vi "GUI Monitoring Graph Selection Window.vi"(14 "OK Button":bool) -> (4 "Graph Selector Out":T1[](array[typedef])=[{"Name"="BPMs Horizontais", "Active"=TRUE}, {"Name"="BPMs Verticais", "Active"=TRUE}, {"Name"="Grupo ACH", "Active"=TRUE}, {"Name"="Grupo ACV", "Active"=TRUE}, {"Name"="Grupo ALV", "Active"=TRUE}] caption="BPMs Horizontais")   [LabVIEW 2011, in "User Interface Window VIs.lvlib"]
uses:
  Types Definitions/Type BPM or PS Selector.ctl
  User Interface Window VIs.lvlib
  Type Definitions.lvlib
panel:
  out "Start plotting?":bool=TRUE
  in  "All/None":bool=TRUE caption="Todos/Nenhum"
  in  "Graph Selector":T1[](array[typedef])=[{"Name"="BPMs Horizontais", "Active"=TRUE}, {"Name"="BPMs Verticais", "Active"=TRUE}, {"Name"="Grupo ACH", "Active"=TRUE}, {"Name"="Grupo ACV", "Active"=TRUE}, {"Name"="Grupo ALV", "Active"=TRUE}] caption="Seleção de Gráficos"
  in  "Cancel Button":bool
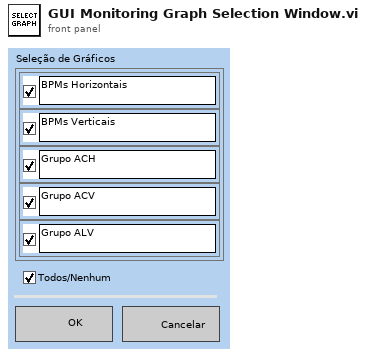
[diagram p1: front panel]
types:
  T1 = typedef "Type Definitions.lvlib/Type BPM or PS Selector.ctl" = cluster{"Name":string, "Active":bool}
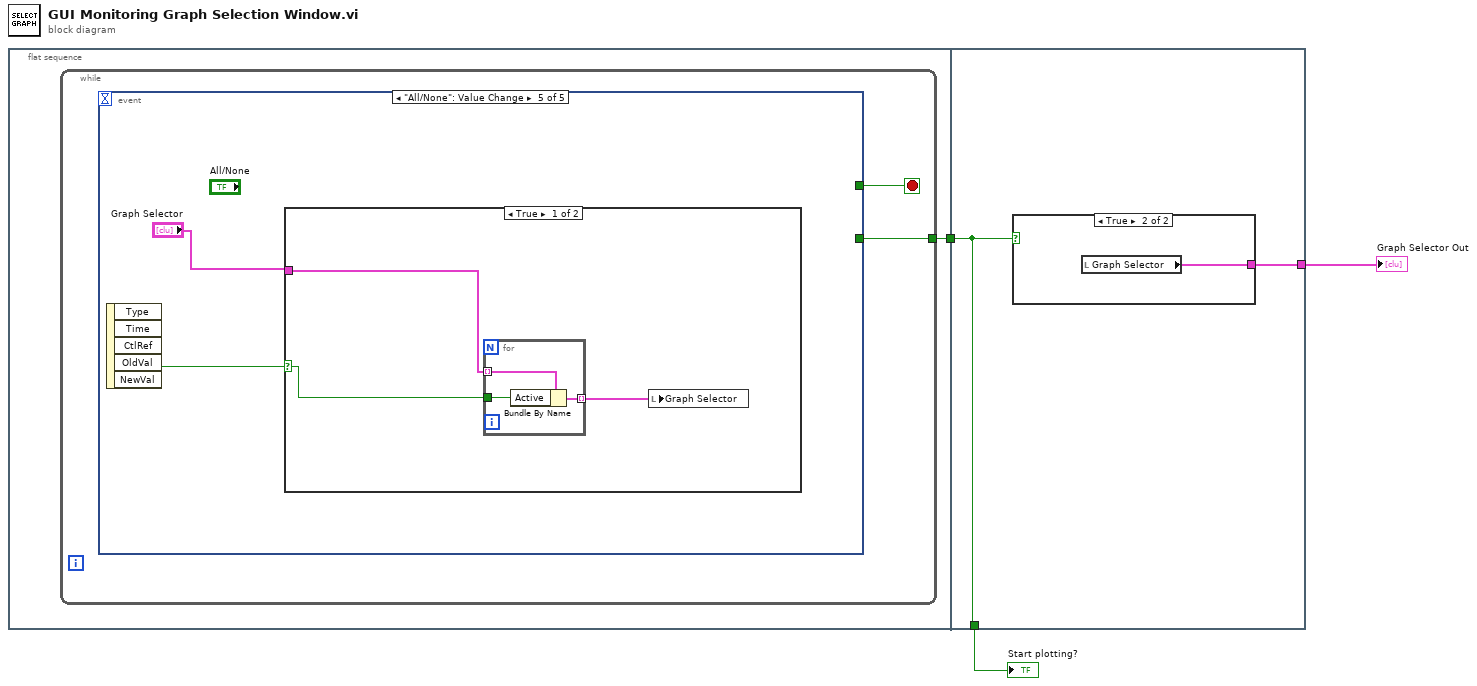
[diagram p0: block diagram]
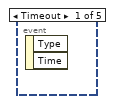
[diagram p2: hidden frame]
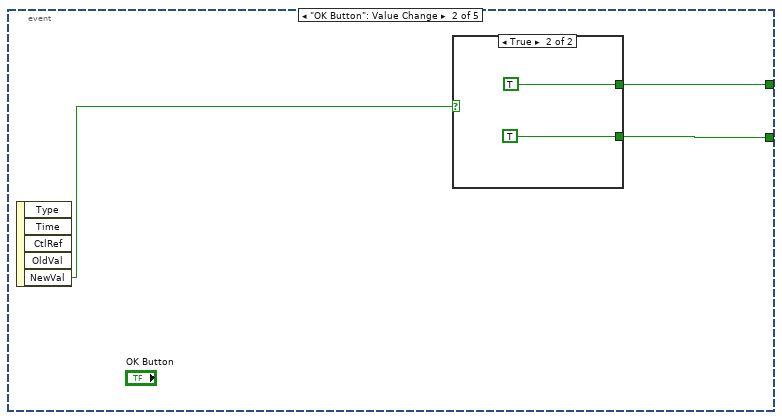
[diagram p3: hidden frame]
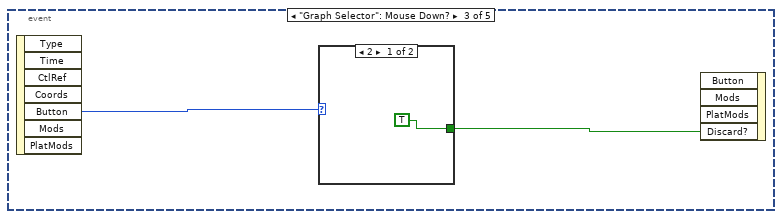
[diagram p5: hidden frame]
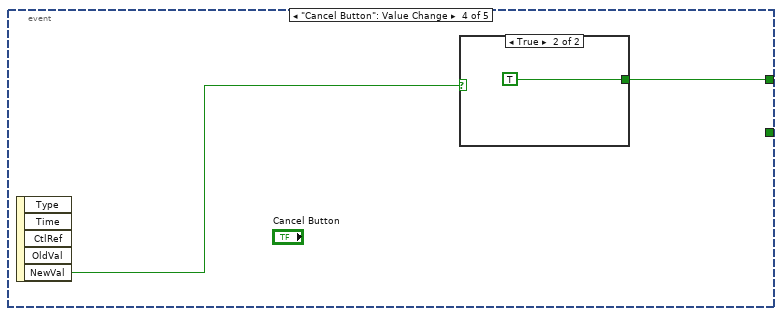
[diagram p7: hidden frame]
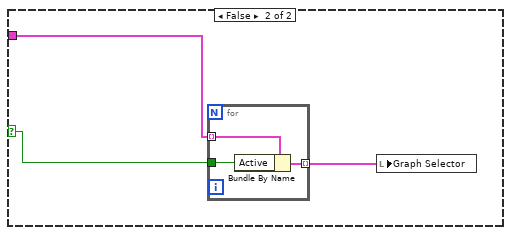
[diagram p9: hidden frame]
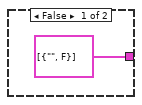
[diagram p10: hidden frame]
diagram:
  n1 = flat-sequence {
    tunnel: [w4] -> w3
    tunnel: w3 -> [w33]
    tunnel: [w33] -> w2
    tunnel: [w32] -> w1
    frame #0 {
      n2 = while {
        tunnel: [w5] -> w4
        stop <- w6 stop-if-true
        n3 = event shown="[4] \"All/None\": Value Change" {
          selector: _ -> [_ _ _ _ _]
          dyn-events: _ -> [_ _ _ _ _]
          timeout: _ -> [_ _ _ _ _]
          tunnel: [_ w9 _ w16 _] -> w6
          tunnel: [_ w8 _ _ _] -> w5
          event Timeout {
            n4 = event-data() -> ()  [unwired: 1 in, 2 out]
          }
          event "OK Button": Value Change {
            n5 = event-data() -> ("NewVal"=w7:bool)  [unwired: 1 in, 4 out]
            n6 = case shown="True" w7 {
              tunnel: [_ TRUE] -> w9
              tunnel: [_ TRUE ("Save and Exit")] -> w8
              frame False {
              }
              frame True {
              }
            }
          }
          event "Graph Selector": Mouse Down? {
            n7 = event-data() -> ("Button"=w13:u16)  [unwired: 1 in, 6 out]
            n8 = case shown="2" w13 {
              tunnel: [TRUE ("Discard?") _] -> w12
              frame 2 {
              }
              frame 1, Default {
              }
            }
            n9 = event-data("Discard?"=w12) -> ()  [unwired: 4 in, 1 out]
          }
          event "Cancel Button": Value Change {
            n10 = event-data() -> ("NewVal"=w15:bool)  [unwired: 1 in, 4 out]
            n11 = case shown="True" w15 {
              tunnel: [_ TRUE] -> w16
              frame False {
              }
              frame True {
              }
            }
          }
          event "All/None": Value Change {
            n12 = event-data() -> ("NewVal"=w19:bool)  [unwired: 1 in, 4 out]
            n13 = case shown="True" w19 {
              selector: w19 -> [w22 w28]
              tunnel: "Graph Selector" -> [w20 w26]
              frame True {
                n14 = for {
                  tunnel: w20 -> [w24] mode=indexing
                  tunnel: [w25] -> w21 mode=indexing
                  tunnel: w22 -> [w23]
                  n15 = Bundle By Name(cluster=w24, "Active"=w23) -> (w25:T1)
                }
                n16 = local write "Graph Selector"(w21) -> ()
              }
              frame False {
                n17 = for {
                  tunnel: w26 -> [w30] mode=indexing
                  tunnel: [w31] -> w27 mode=indexing
                  tunnel: w28 -> [w29]
                  n18 = Bundle By Name(cluster=w30, "Active"=w29) -> (w31:T1)
                }
                n19 = local write "Graph Selector"(w27) -> ()
              }
            }
          }
        }
      }
    }
    frame #1 {
      n20 = case shown="True" w33 {
        tunnel: [T1[] [{"Name"="", "Active"=FALSE}] ("BPM Graph Selector Horizontal") w35] -> w32
        frame False {
        }
        frame True {
          n21 = local read "Graph Selector"() -> (w35:T1[])
        }
      }
    }
  }
  "Start plotting?" <- w2
  "Graph Selector Out" <- w1
